vi "VI Tree.vi"   [LabVIEW 2016, in "Agilent E4980.lvlib"]
doc: "This is the instrument driver for the Agilent E4980. The VI Tree displays all the user-callable VIs of the instrument driver in an organized table."
uses:
  <instrlib>/Agilent E4980/Agilent E4980.lvlib
  <instrlib>/Agilent E4980/Public/Action-Status/Clear Comparator Bin (Limit).vi
  <instrlib>/Agilent E4980/Public/Utility/Configure System (Display).vi
  <instrlib>/Agilent E4980/Public/Data/Low Level/Read Functional Data (AC Monitor).vi
panel:
  # "(c) 2007-2015 National Instruments.  ALL RIGHTS RESERVED."
  # "SEE DIAGRAM\nFOR VI TREE."
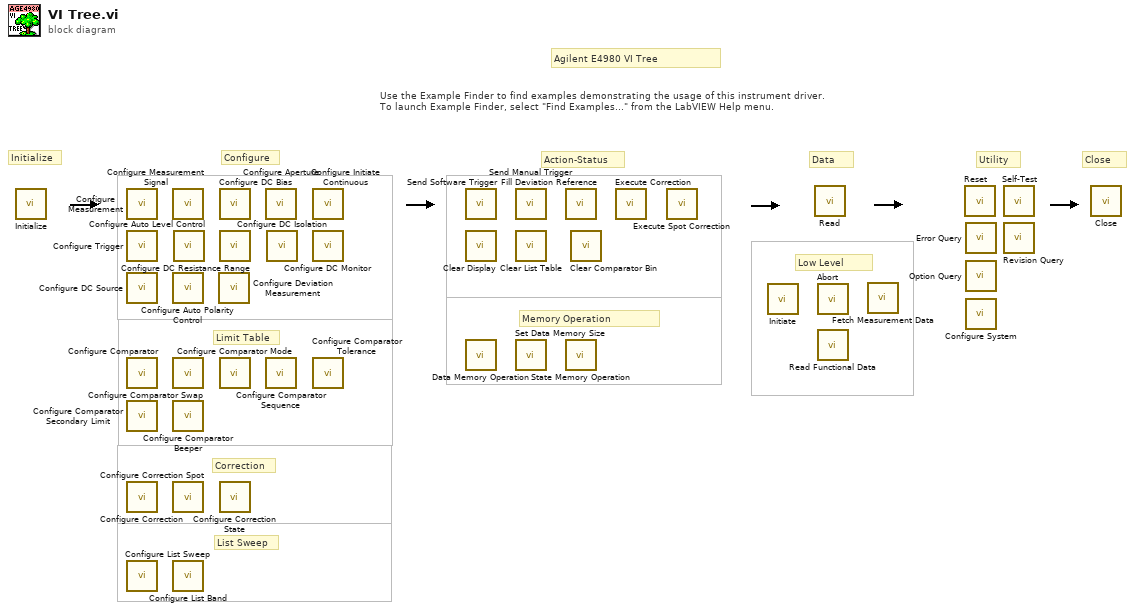
[diagram p0: block diagram]
diagram:
  # "Data"
  # "Low Level"
  # "Memory Operation"
  # "List Sweep"
  # "Correction"
  # "Limit Table"
  # "Close"
  # "Utility"
  # "Action-Status"
  # "Configure"
  # "Initialize"
  # "Agilent E4980 VI Tree"
  # "Use the Example Finder to find examples demonstrating the usage of this instrument driver.\nTo launch Example Finder, select \"Find Examples...\" from the LabVIEW Help menu."
  n1 = call <instrlib>:"Initialize.vi"() -> ()  [unwired: 10 in, 2 out]
  n2 = call <instrlib>:"Configure Measurement.vi"() -> ()  [unwired: 10 in, 2 out]
  n3 = call <instrlib>:"Configure Trigger.vi"() -> ()  [unwired: 10 in, 2 out]
  n4 = call <instrlib>:"Configure DC Source.vi"() -> ()  [unwired: 10 in, 2 out]
  n5 = call <instrlib>:"Configure Comparator.vi"() -> ()  [unwired: 10 in, 2 out]
  n6 = call <instrlib>:"Configure Comparator Secondary Limit.vi"() -> ()  [unwired: 10 in, 2 out]
  n7 = call <instrlib>:"Configure Correction.vi"() -> ()  [unwired: 10 in, 2 out]
  n8 = call <instrlib>:"Configure List Sweep.vi"() -> ()  [unwired: 10 in, 2 out]
  n9 = call <instrlib>:"Configure Measurement Signal.vi"() -> ()  [unwired: 10 in, 2 out]
  n10 = call <instrlib>:"Configure Auto Polarity Control.vi"() -> ()  [unwired: 10 in, 2 out]
  n11 = call <instrlib>:"Configure Comparator Swap.vi"() -> ()  [unwired: 10 in, 2 out]
  n12 = call <instrlib>:"Configure Comparator Beeper.vi"() -> ()  [unwired: 10 in, 2 out]
  n13 = call <instrlib>:"Configure Correction Spot.vi"() -> ()  [unwired: 10 in, 2 out]
  n14 = call <instrlib>:"Configure List Band.vi"() -> ()  [unwired: 10 in, 2 out]
  n15 = call <instrlib>:"Configure Auto Level Control.vi"() -> ()  [unwired: 10 in, 2 out]
  n16 = call <instrlib>:"Configure Deviation Measurement.vi"() -> ()  [unwired: 10 in, 2 out]
  n17 = call <instrlib>:"Configure DC Bias.vi"() -> ()  [unwired: 10 in, 2 out]
  n18 = call <instrlib>:"Configure DC Resistance Range.vi"() -> ()  [unwired: 10 in, 2 out]
  n19 = call <instrlib>:"Configure Comparator Mode.vi"() -> ()  [unwired: 10 in, 2 out]
  n20 = call <instrlib>:"Configure Correction State.vi"() -> ()  [unwired: 10 in, 2 out]
  n21 = call <instrlib>:"Configure Aperture.vi"() -> ()  [unwired: 10 in, 2 out]
  n22 = call <instrlib>:"Configure Comparator Sequence.vi"() -> ()  [unwired: 10 in, 2 out]
  n23 = call <instrlib>:"Configure DC Isolation.vi"() -> ()  [unwired: 10 in, 2 out]
  n24 = call <instrlib>:"Configure Initiate Continuous.vi"() -> ()  [unwired: 10 in, 2 out]
  n25 = call <instrlib>:"Configure DC Monitor.vi"() -> ()  [unwired: 10 in, 2 out]
  n26 = call <instrlib>:"Configure Comparator Tolerance.vi"() -> ()  [unwired: 10 in, 2 out]
  n27 = call <instrlib>:"Send Software Trigger.vi"() -> ()  [unwired: 10 in, 2 out]
  n28 = call <instrlib>:"Clear Display.vi"() -> ()  [unwired: 10 in, 2 out]
  n29 = call <instrlib>:"Data Memory Operation.vi"() -> ()  [unwired: 10 in, 2 out]
  n30 = call <instrlib>:"Send Manual Trigger.vi"() -> ()  [unwired: 10 in, 2 out]
  n31 = call <instrlib>:"Clear List Table.vi"() -> ()  [unwired: 10 in, 2 out]
  n32 = call <instrlib>:"Set Data Memory Size.vi"() -> ()  [unwired: 10 in, 2 out]
  n33 = call <instrlib>:"Fill Deviation Reference.vi"() -> ()  [unwired: 10 in, 2 out]
  n34 = call <instrlib>:"State Memory Operation.vi"() -> ()  [unwired: 10 in, 2 out]
  n35 = call-poly <instrlib>:"Clear Comparator Bin.vi"() -> ()  [unwired: 10 in, 2 out]
  n36 = call <instrlib>:"Execute Correction.vi"() -> ()  [unwired: 10 in, 2 out]
  n37 = call <instrlib>:"Execute Spot Correction.vi"() -> ()  [unwired: 10 in, 2 out]
  n38 = call <instrlib>:"Initiate.vi"() -> ()  [unwired: 10 in, 2 out]
  n39 = call <instrlib>:"Read.vi"() -> ()  [unwired: 8 in, 4 out]
  n40 = call <instrlib>:"Abort.vi"() -> ()  [unwired: 10 in, 2 out]
  n41 = call-poly <instrlib>:"Read Functional Data.vi"() -> ()  [unwired: 8 in, 4 out]
  n42 = call <instrlib>:"Fetch Measurement Data.vi"() -> ()  [unwired: 7 in, 5 out]
  n43 = call <instrlib>:"Reset.vi"() -> ()  [unwired: 10 in, 2 out]
  n44 = call <instrlib>:"Error Query.vi"() -> ()  [unwired: 8 in, 4 out]
  n45 = call <instrlib>:"Option Query.vi"() -> ()  [unwired: 9 in, 3 out]
  n46 = call-poly <instrlib>:"Configure System.vi"() -> ()  [unwired: 10 in, 2 out]
  n47 = call <instrlib>:"Self-Test.vi"() -> ()  [unwired: 8 in, 4 out]
  n48 = call <instrlib>:"Revision Query.vi"() -> ()  [unwired: 8 in, 4 out]
  n49 = call <instrlib>:"Close.vi"() -> ()  [unwired: 11 in, 1 out]
